vi "Hexapod_GUI_2.vi"(11 "GUI_cluster":T1={"Sub Panel"=refnum, "GUIdevice"="Bella_LP_Mode", "CtlRef"=refnum, "user event out"=refnum}) -> ()   [LabVIEW 2011]
uses:
  GUI_Template/GUI_master/tcp_new_data_event.ctl
  GUI_Template/GUI_master/tcp new data cluster.ctl
  Controls/GUI_cluster.ctl
  Controls/eventtypdef.ctl
panel:
  in  "<command>::1":bool
  in  "stepsize::1":dbl caption="stepsize" min=0.0 max=10.0
  in  "relativemove.zpos::1":bool
  in  "relativemove.zneg::1":bool
  in  "wpos::1":dbl caption="w"
  in  "vpos::1":dbl caption="v"
  in  "upos::1":dbl caption="u"
  in  "zpos::1":dbl caption="z" min=-12.0 max=12.0
  in  "ypos::1":dbl caption="y" min=-20.0 max=20.0
  in  "xpos::1":dbl caption="x" min=-20.0 max=20.0
  in  "relativemove.ypos::1":bool
  in  "relativemoveyneg::1":bool
  in  "relativemove.xneg::1":bool
  in  "relativemove.xpos::1":bool
  out "tcp data event":T2
  out "GUIdevice 1":string="Bella_LP_Mode"
  in  "stop":bool
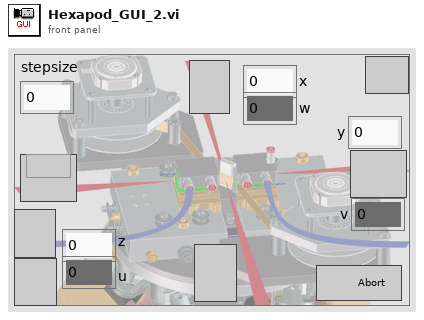
[diagram p1: front panel]
types:
  T1 = typedef "GUI_cluster.ctl" = cluster{"Sub Panel":refnum<vi>, "GUIdevice":string, "CtlRef":refnum<vi>, "user event out":refnum<user-event>}
  T2 = typedef "tcp_new_data_event.ctl" = refnum<user-event>
  T3 = typedef "eventtypdef.ctl" = cluster{"label":string, "Sub Panel":refnum<vi>, "CtlRef":refnum<vi>, "This VI":refnum<vi>}
  T4 = typedef "tcp new data cluster.ctl" = cluster{"EventEnum":enum16{"new data", "connection status update"}, "Device name":string}
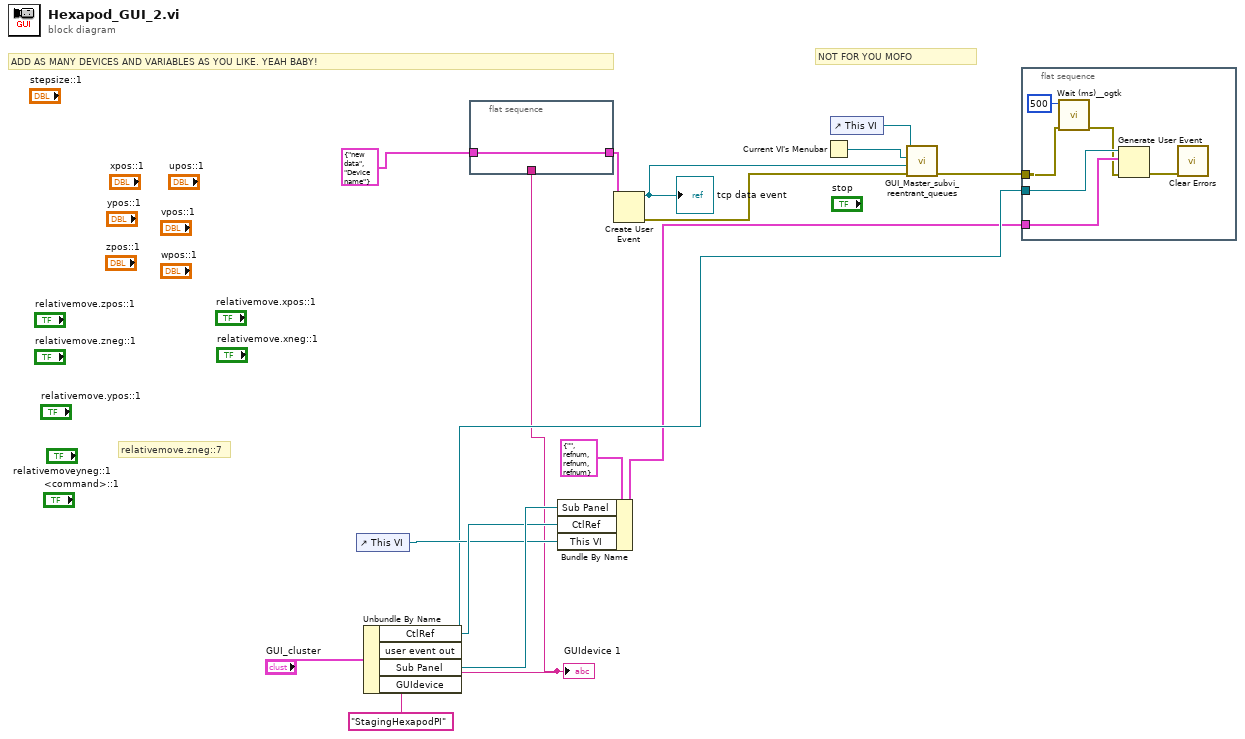
[diagram p0: block diagram]
diagram:
  w1 = "StagingHexapodPI" ("GUIdevice")
  # "relativemove.zneg::7"
  # "ADD AS MANY DEVICES AND VARIABLES AS YOU LIKE. YEAH BABY!"
  # "NOT FOR YOU MOFO"
  n1 = control-ref of="This VI"() -> (w5:refnum<vi>)
  n2 = Unbundle By Name("GUI_cluster") -> ("CtlRef"=w6:refnum<vi>, "user event out"=w3:refnum<user-event>, "Sub Panel"=w9:refnum<vi>)  [unwired: 1 out]
  n3 = flat-sequence {
    tunnel: T4 {"EventEnum"=enum."new data", "Device name"="Device name"} ("New Event") -> [w16]
    tunnel: [w16] -> w7
    tunnel: w1 -> [_]
    frame #0 {
    }
  }
  n4 = Bundle By Name(cluster=T3 {"label"="", "Sub Panel"=refnum, "CtlRef"=refnum, "This VI"=refnum} ("event data"), "Sub Panel"=w9, "CtlRef"=w6, "This VI"=w5) -> (w2:T3)
  n5 = Create User Event(user event datatype=w7) -> (user event=w12:refnum<user-event>, error out=w13:errorcluster)  [unwired: 1 in]
  "tcp data event" <- w12
  n6 = Current VI's Menubar() -> (w14:refnum<k9>)
  n7 = control-ref of="This VI"() -> (w15:refnum<vi>)
  n8 = call "GUI_Master_subvi_reentrant_queues.vi"("error in (no error)"=w13, "tcp data event"=w12, "Caller menu reference"=w14, "Caller VI ref"=w15) -> ("error out"=w4:errorcluster)  [unwired: 7 in]
  n9 = flat-sequence {
    tunnel: w4 -> [w19]
    tunnel: w3 -> [w22]
    tunnel: w2 -> [w21]
    frame #0 {
      n10 = call <userlib>:"Wait (ms)__ogtk.vi"("error in (no error)"=w19, "milliseconds to wait"=u32 500) -> ("error out"=w18:errorcluster)  [unwired: 8 in, 1 out]
      n11 = Generate User Event(user event=w22, event data cluster=w21, error in=w18) -> (error out=w20:errorcluster)  [unwired: 1 out]
      n12 = call <vilib>:"Clear Errors.vi"("error in (no error)"=w20) -> ()  [unwired: 6 in, 1 out]
    }
  }
  "GUIdevice 1" <- w1
